vi "UI.vi"() -> ()   [LabVIEW 2017]
panel:
  out "Chart":dbl(graph)
  in  "Slider":dbl(slide) scale=0.0..10.0
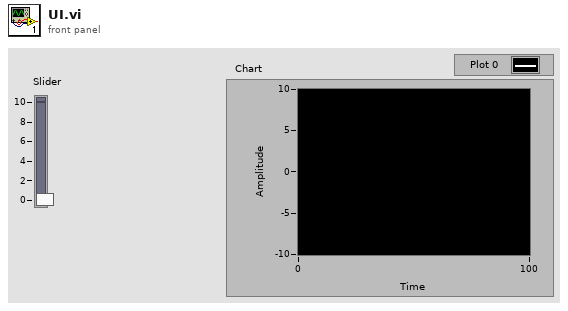
[diagram p1: front panel]
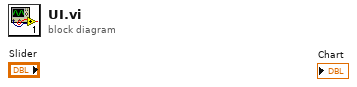
[diagram p0: block diagram]
diagram:
